vi "Perform_Meas_Setup.vi"(2 "Simulate/Run":T1, 3 "String array":string[](array[string])) -> (0 "Continue?":bool, 1 "FFID Bkgnd needed?":bool)   [LabVIEW 2022 SP3]
uses:
  Controls/User_Specific_mode.ctl
  Controls/Setup.ctl
  Controls/Save_Data.ctl
  Camera Server/Camera enum/Camera resolution.ctl
  <vilib>/Utility/error.llb/Trim Whitespace One-Sided.vi
  Globals/LDA_global.vi
  Globals/Dynamic_call_global.ph.vi
  Globals/Meas_global.vi
  Controls/Inst_type.ctl
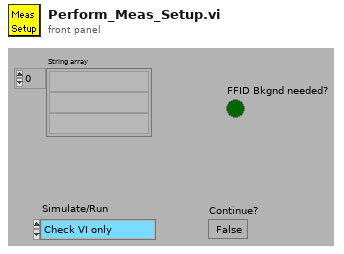
[diagram p1: front panel]
types:
  T1 = typedef "User_Specific_mode.ctl" = enum16{"Check VI only", "Run VI"}
  T2 = typedef "Save_Data.ctl" = enum16{"Save No Data", "Save Data"}
  T3 = typedef "Setup.ctl" = enum16{"Run Program", "Show Setup", "Save Current Setup", "Setup Front Panel"}
  T4 = typedef "Inst_type.ctl" = enum16{"Raw voltage", "Raw with zero offsetting", "Propeller anemometer", "Pressure Transducer", "Pitot-static tube", "Hot wire", "Cross wire 1", "Cross wire 2", "Generic Linear", "Generic Polynomial", "Generic BackPoly", "Fast FID", "Thermocouple", "Cold wire", "Pulsed Wire", "LDA Vel", "LDA Tran time", "LDA Arr time", "Microphone"}
  T5 = typedef "Camera resolution.ctl" = u8
  T6 = typedef "LDA_Channel.ctl" = cluster{"Wavelength (nm)":dbl, "Vel Comp":string, "Max Velocity":dbl, "Min Velocity":dbl, "Max Record length":u16, "Signal gain (dB)":i16, "High voltage":i16, "Optics Conversion Factor":dbl, "Min Record length":u16, "Multiply Velocity by -1":bool, "Signal to Noise Ratio":string, "Validation Ratio":string, "Probe":string, "Laser":string, "BSA":string, "Lense":string, "Beam Separation (mm)":dbl, "Focal Length (mm)":dbl, "COLOUR":u32, "BSA IP":string, "Velocity Range (m/s)":dbl, "Centre Velocity (m/s)":dbl, "Unshifted mW":dbl, "Shifted mW":dbl, "Bandwidth Hz":dbl, "Req Sampling Rate Hz":dbl, "Ch":i32, "CenterFreq Hz":dbl, "Laser IP":string, "Sync Delay (s)":dbl}
  T7 = typedef "Analysis_info_cluster.ctl" = cluster{"Colour":u32, "Inst type":T4, "Inst name":string, "Symbol":string, "Code name":string, "Extra Info":string, "Inst Array":T8, "U":dbl, "u^2":dbl, "u^3":dbl, "u^4":dbl, "Skew_u":dbl, "Kurt_u":dbl, "Sd Error in Mean":dbl, "% u'/U":dbl, "X":dbl, "Y":dbl, "Z":dbl, "Timescale integral Estimate":dbl, "Sd Error in Variance":dbl, "Calib File":path, "Calib Constants":dbl[], "Output Position":bool, "Stats":enum16{"None", "Basic", "Full"}, "Av Sampling Rate":dbl, "Av No of Samples":dbl, "Total Meas Time (s)":dbl, "OrigChName":string, "Max value":dbl, "Min value":dbl, "Req Sample Rate Hz":dbl, "Sync Delay Time (s)":dbl, "Ch No":i16, "Device":string, "Use Latest Calib":bool, "Port":string, "Metadata Ch Names":string[], "Metadata Ch Values":string[], "Label":string, "chState":T9, "Point Drift":dbl, "inputConfig":string}
  T8 = typedef "Instrument_Array.ctl" = enum16{"PWA", "LDA", "Analogue"}
  T9 = typedef "channelState.ctl" = enum32{"No Selection", "Solo", "Mute"}
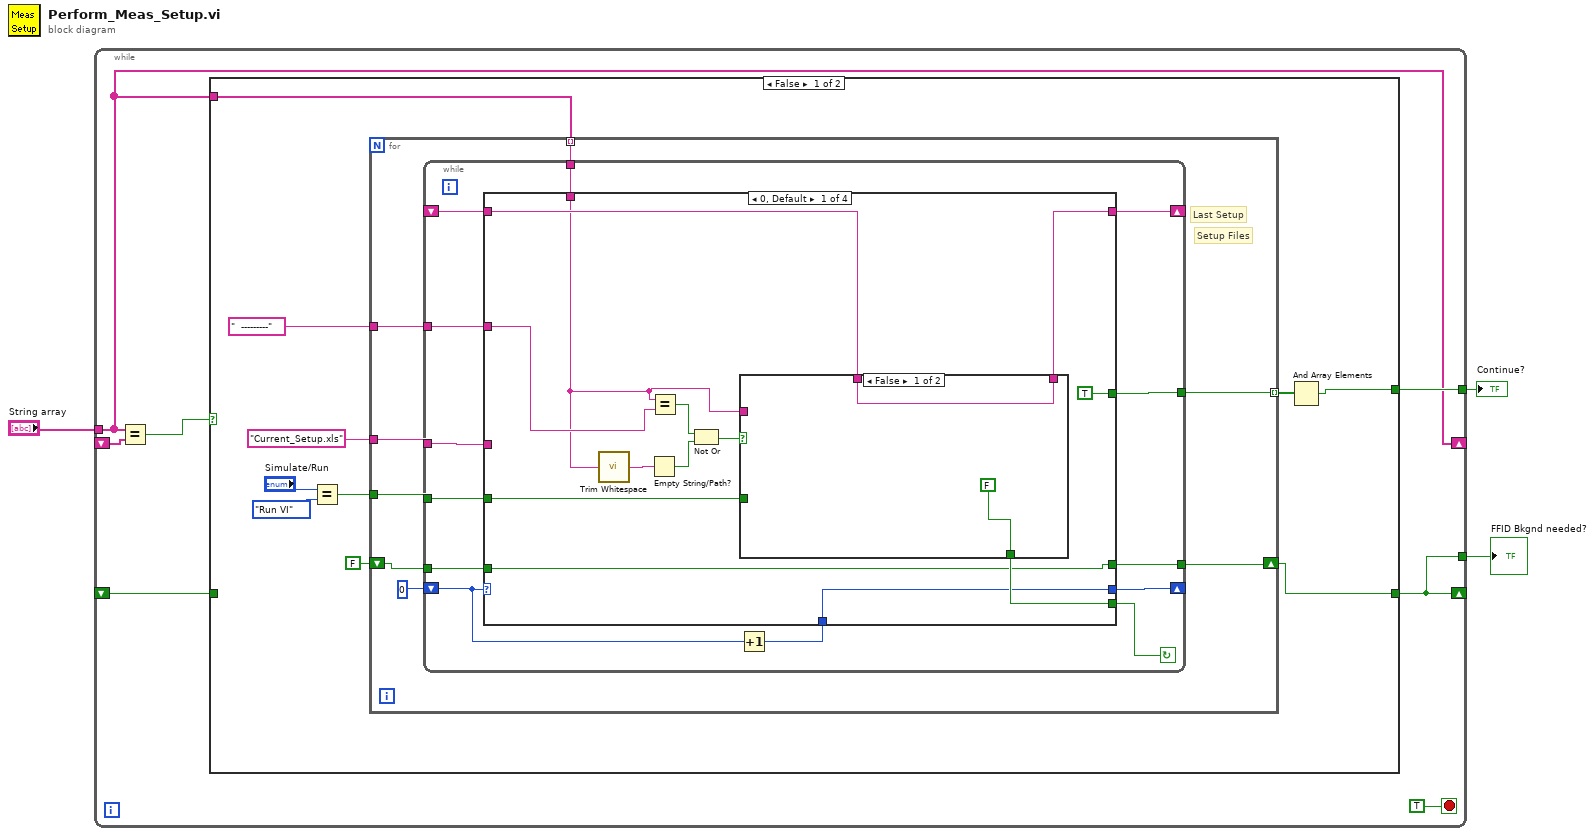
[diagram p0: block diagram]
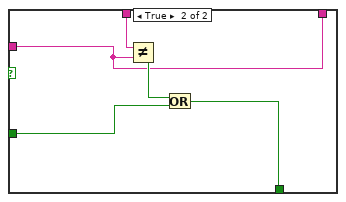
[diagram p2: hidden frame]
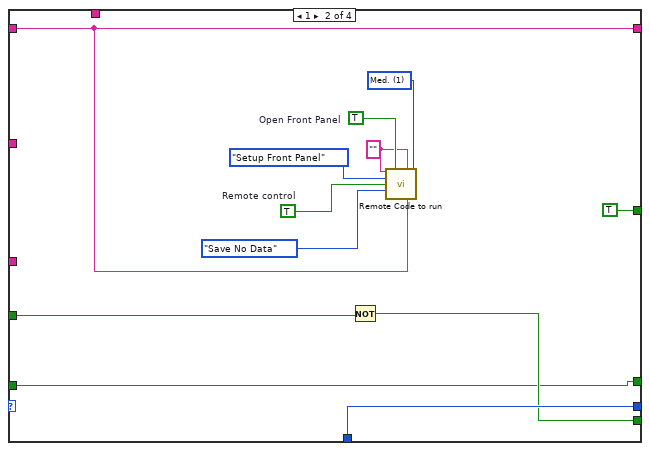
[diagram p3: hidden frame]
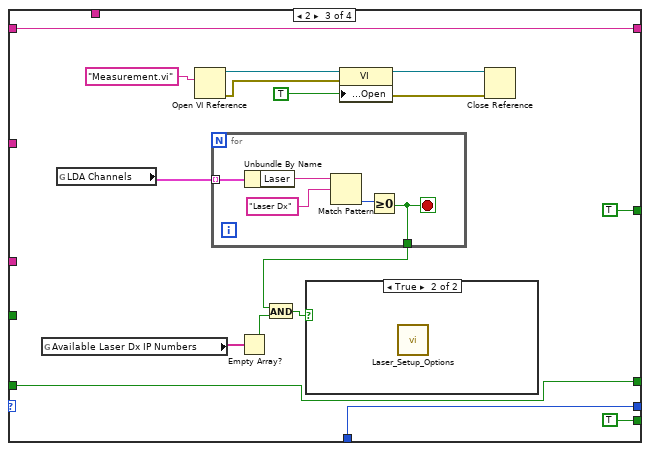
[diagram p4: hidden frame]
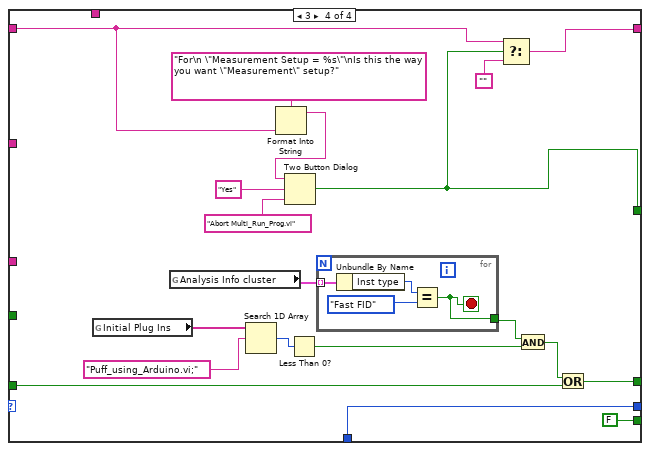
[diagram p6: hidden frame]
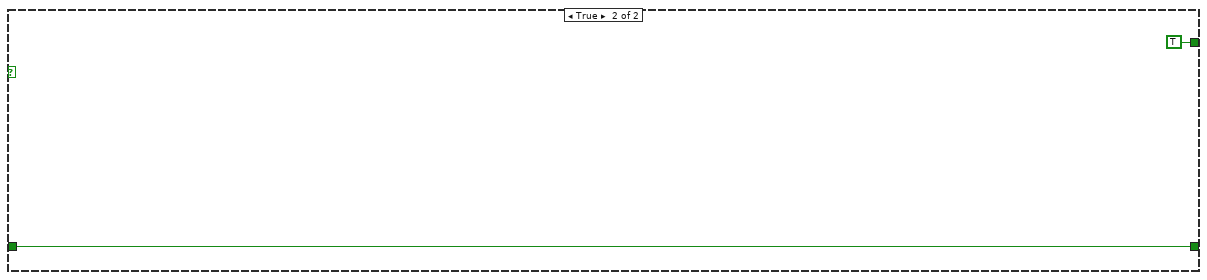
[diagram p7: hidden frame]
diagram:
  n1 = while {
    tunnel: [w10] -> w3
    tunnel: [w4] -> w2
    shift-right: [w6] -> _
    shift-left: _ -> [w8]
    tunnel: "String array" -> [w6]
    shift-right: [w4] -> _
    shift-left: _ -> [w5]
    stop <- TRUE stop-if-true
    n2 = Equal?(x=w6, y=w8) -> (x = y?=w7:bool)
    n3 = case shown="False" w7 {
      tunnel: [w13 TRUE] -> w10
      tunnel: [w11 w118] -> w4
      tunnel: w6 -> [w12 _]
      tunnel: w5 -> [_ w118]
      frame False {
        n4 = Equal?(x="Simulate/Run", y=User_Specific_mode."Run VI" ("Simulate/Run")) -> (x = y?=w17:bool)
        n5 = for {
          tunnel: "Current_Setup.xls" ("name or relative path") -> [w27]
          tunnel: w17 -> [w26]
          tunnel: w12 -> [w25] mode=indexing
          tunnel: [w24] -> w16 mode=indexing
          tunnel: "  ---------" ("f") -> [w23]
          shift-right: [w21] -> w11
          shift-left: FALSE -> [w22]
          # "Last Setup"
          # "Setup Files"
          n6 = while {
            tunnel: w26 -> [w33]
            tunnel: w27 -> [w34]
            shift-left: _ -> [w36]
            shift-right: [w35] -> _
            tunnel: [w37] -> w24
            shift-left: 0 -> [w40]
            shift-right: [w38] -> _
            tunnel: w25 -> [w32]
            tunnel: w23 -> [w31]
            tunnel: w22 -> [w30]
            tunnel: [w29] -> w21
            stop <- w41 continue-if-true
            n7 = Increment(x=w40) -> (x+1=w39:i32)
            n8 = case shown="0, Default" w40 {
              tunnel: [w51 w68 TRUE FALSE] -> w41
              tunnel: w39 -> [w49 w70 w89 w113]
              tunnel: [w49 w70 w89 w113] -> w38
              tunnel: [TRUE ("T button?") TRUE ("T button?") TRUE ("T button?") w107] -> w37
              tunnel: w36 -> [w53 w65 w88 w105]
              tunnel: [w52 w65 w88 w106] -> w35
              tunnel: w34 -> [_ _ _ _]
              tunnel: w33 -> [w50 w69 _ _]
              tunnel: w32 -> [w44 _ _ _]
              tunnel: w31 -> [w45 _ _ _]
              tunnel: w30 -> [w42 w62 w74 w96]
              tunnel: [w42 w62 w74 w95] -> w29
              frame 0, Default {
                n9 = call <vilib>:"Trim Whitespace.vi"("string"=w44) -> ("trimmed string"=w43:string)  [unwired: 1 in]
                n10 = Empty String/Path?(string/path=w43) -> (empty?=w47:bool)
                n11 = Equal?(x=w44, y=w45) -> (x = y?=w48:bool)
                n12 = Not Or(1:w47, 2:w48) -> (0:w46:bool)
                n13 = case shown="False" w46 {
                  tunnel: [w56 w58] -> w52
                  tunnel: w44 -> [_ w58]
                  tunnel: w53 -> [w56 w61]
                  tunnel: [FALSE w59] -> w51
                  tunnel: w50 -> [_ w57]
                  frame False {
                  }
                  frame True {
                    n14 = Not Equal?(x=w61, y=w58) -> (x != y?=w60:bool)
                    n15 = Or(x=w60, y=w57) -> (x .or. y?=w59:bool)
                  }
                }
              }
              frame 1 {
                w63 = T5 1 items=["Low", "Med.", "High", "Max."] ("Camera Resolution")
                w64 = "" ("Extra command String")
                w72 = TRUE  # Remote control
                w73 = TRUE  # Open Front Panel
                n16 = Not(x=w69) -> (.not. x?=w68:bool)
                n17 = call "Remote Code to run.vi"("Extra command String"=w64, "Open Front Panel"=w73, "Current Row Comments"=w64, "Camera Resolution"=w63, "setup"=Setup."Setup Front Panel", "Remote control"=w72, "File"=Save_Data."Save No Data", "Setup filename"=w65) -> ()  [unwired: 7 in, 1 out]
              }
              frame 2 {
                n18 = global read "LDA_global.vi" "Available Laser Dx IP Numbers"() -> (w78:string[])
                n19 = global read "LDA_global.vi" "LDA Channels"() -> (w79:T6[])
                n20 = Open VI Reference(vi path="Measurement.vi") -> (vi reference=w84:refnum<vi>, error out=w85:errorcluster)  [unwired: 1 in, 4 out]
                n21 = for {
                  tunnel: w79 -> [w94] mode=indexing
                  tunnel: [w90] -> w75
                  stop <- w90 stop-if-true
                  n22 = Unbundle By Name(w94) -> ("Laser"=w93:string)
                  n23 = Match Pattern(string=w93, regular expression="Laser Dx") -> (offset past match=w91:i32)  [unwired: 1 in, 3 out]
                  n24 = Greater Or Equal To 0?(x=w91) -> (x >= 0?=w90:bool)
                }
                n25 = Empty Array?(array=w78) -> (empty?=w77:bool)
                n26 = And(x=w75, y=w77) -> (x .and. y?=w76:bool)
                n27 = case shown="True" w76 {
                  frame False {
                  }
                  frame True {
                    n28 = call "Laser_Setup_Options.vi"() -> ()  [unwired: 5 in, 4 out]
                  }
                }
                n29 = property class="VI"(reference=w84, error in=w85, "Front Panel Window:Open"=TRUE) -> (reference out=w82:refnum<vi>, error out=w81:errorcluster)
                n30 = Close Reference(reference=w82, error in (no error)=w81) -> ()  [unwired: 1 out]
              }
              frame 3 {
                n31 = global read "Dynamic_call_global.ph.vi" "Initial Plug Ins"() -> (w103:string[])
                n32 = global read "Meas_global.vi" "Analysis Info cluster"() -> (w101:T7[])
                n33 = Search 1D Array(1D array=w103, element="Puff_using_Arduino.vi;") -> (index of element=w100:i32)  [unwired: 1 in]
                n34 = Format Into String(format string="For\n \"Measurement Setup = %s\"\nIs this the way you want \"Measurement\" setup?" ("message"), w105) -> (resulting string=w112:string)  [unwired: 2 in, 1 out]
                n35 = Two Button Dialog(message=w112, 1:"Abort Multi_Run_Prog.vi" ("F button name (\"Cancel\")"), 2:"Yes" ("T button name (\"OK\")")) -> (T button?=w107:bool)
                n36 = Less Than 0?(x=w100) -> (x < 0?=w98:bool)
                n37 = for {
                  tunnel: w101 -> [w117] mode=indexing
                  tunnel: [w114] -> w99
                  stop <- w114 stop-if-true
                  n38 = Unbundle By Name(w117) -> ("Inst type"=w116:T4)
                  n39 = Equal?(x=w116, y=Inst_type."Fast FID" ("Inst type")) -> (x = y?=w114:bool)
                }
                n40 = Select(t=w105, s=w107, f="") -> (s? t:f=w106:string)
                n41 = And(x=w99, y=w98) -> (x .and. y?=w97:bool)
                n42 = Or(x=w97, y=w96) -> (x .or. y?=w95:bool)
              }
            }
          }
        }
        n43 = And Array Elements(Boolean array=w16) -> (logical AND=w13:bool)
      }
      frame True {
      }
    }
  }
  "Continue?" <- w3
  "FFID Bkgnd needed?" <- w2
